vi "Sign Extend Variable Bit Number.vi"(7 "Variable Bit Number":bool[](array[boolean])) -> (8 "Sign extended value":dbl format="%#.6f")   [LabVIEW 2013, in "AIT 664 Custom Device.lvlib"]
uses:
  AIT 664 Custom Device.lvlib
panel:
  out "Number of Bits":i32=3
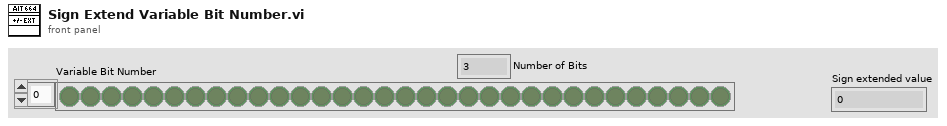
[diagram p1: front panel]
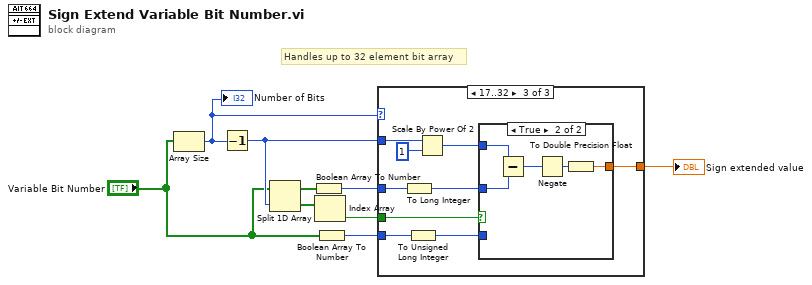
[diagram p0: block diagram]
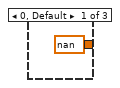
[diagram p2: hidden frame]
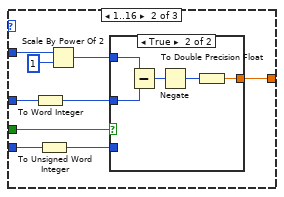
[diagram p3: hidden frame]
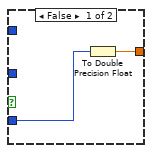
[diagram p4: hidden frame]
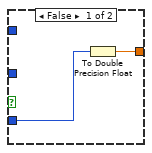
[diagram p5: hidden frame]
diagram:
  # "Handles up to 32 element bit array"
  n1 = Array Size(array="Variable Bit Number") -> (size(s)=w1:i32)
  "Number of Bits" <- w1
  n2 = Decrement(x=w1) -> (x-1=w3:i32)
  n3 = Split 1D Array(array="Variable Bit Number", index=w3) -> (first subarray=w7:bool[], second subarray=w8:bool[])
  n4 = Boolean Array To Number(Boolean array=w7) -> (number=w6:u32)
  n5 = Index Array(array=w8) -> (element=w9:bool)  [unwired: 1 in]
  n6 = Boolean Array To Number(Boolean array="Variable Bit Number") -> (number=w4:u32)
  n7 = case shown="17..32" w1 {
    tunnel: w9 -> [_ w19 w35]
    tunnel: w6 -> [_ w16 w32]
    tunnel: [nan w14 w30] -> w5
    tunnel: w4 -> [_ w13 w29]
    tunnel: w3 -> [_ w11 w27]
    frame 0, Default {
    }
    frame 1..16 {
      n8 = To Word Integer(number=w16) -> (16bit integer=w15:i16)
      n9 = To Unsigned Word Integer(number=w13) -> (unsigned 16bit integer=w12:u16)
      n10 = Scale By Power Of 2(n=w11, x=i16 1 ("index")) -> (x*2^n=w17:i16)
      n11 = case shown="True" w19 {
        tunnel: w17 -> [_ w26]
        tunnel: w15 -> [_ w25]
        tunnel: [w20 w22] -> w14
        tunnel: w12 -> [w21 _]
        frame False {
          n12 = To Double Precision Float(number=w21) -> (double precision float=w20:dbl)
        }
        frame True {
          n13 = Subtract(x=w26, y=w25) -> (x-y=w24:i16)
          n14 = Negate(x=w24) -> (-x=w23:i16)
          n15 = To Double Precision Float(number=w23) -> (double precision float=w22:dbl)
        }
      }
    }
    frame 17..32 {
      n16 = To Long Integer(number=w32) -> (32bit integer=w31:i32)
      n17 = To Unsigned Long Integer(number=w29) -> (unsigned 32bit integer=w28:u32)
      n18 = Scale By Power Of 2(n=w27, x=1 ("index")) -> (x*2^n=w33:i32)
      n19 = case shown="True" w35 {
        tunnel: w33 -> [_ w42]
        tunnel: w31 -> [_ w41]
        tunnel: [w36 w39] -> w30
        tunnel: w28 -> [w37 _]
        frame False {
          n20 = To Double Precision Float(number=w37) -> (double precision float=w36:dbl)
        }
        frame True {
          n21 = Subtract(x=w42, y=w41) -> (x-y=w38:i32)
          n22 = Negate(x=w38) -> (-x=w40:i32)
          n23 = To Double Precision Float(number=w40) -> (double precision float=w39:dbl)
        }
      }
    }
  }
  "Sign extended value" <- w5
